vi "Pre Launch Init.vi"(11 "Island Watch in":refnum<class "Island Watch.lvclass">) -> (0 "error out":errorcluster, 3 "Island Watch out":refnum<class "Island Watch.lvclass">)   [LabVIEW 2015, in "Island Watch Actor.lvlib" / "Island Watch.lvclass"]
doc: "(<B>Filename</B>: Actor Framework.lvlib:Actor.lvclass:Pre Launch Init.vi)\n\nDefines behavior that occurs after the Launch Nested Actor method is invoked but before the actor's Actor Core method begins running.\n\nBy default, this method does nothing. A descendant class may override it to define behavior."
uses:
  Island Watch.lvclass
  Island Watch.lvclass/Island Watch.ctl
  <vilib>/ActorFramework/Actor/Actor.lvclass
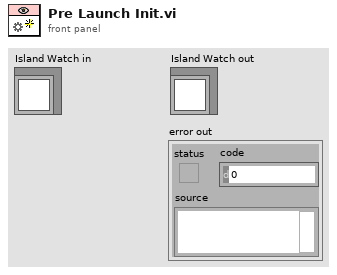
[diagram p1: front panel]
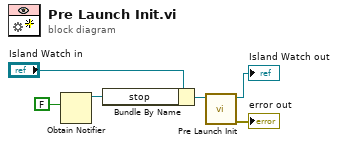
[diagram p0: block diagram]
diagram:
  n1 = Obtain Notifier(notification data type=FALSE) -> (notifier out=w2:refnum<notifier>)  [unwired: 3 in, 2 out]
  n2 = Bundle By Name(cluster="Island Watch in", "stop"=w2) -> (w3:refnum<class "Island Watch.lvclass">)
  n3 = call-parent "Pre Launch Init.vi"("Actor in"=w3) -> ("error out"=→"error out":errorcluster, "Actor out"=→"Island Watch out":refnum<class "Island Watch.lvclass">)  [unwired: 9 in]
